vi "SetAnalogTrigger.vi"(8 "error in (no error)":errorcluster, 10 "Trigger Config":T1={"Channel"=enum."chn B", "Edge"=0, "Level[V]"=0.5} {"Edge" items=["RISING", "FALLING", "ANY"]}, 11 "reference in":refnum<k24>) -> (0 "error out":errorcluster, 3 "reference out":refnum<k24>)   [LabVIEW 2019, in "LabNation Scope Driver.lvlib"]
doc: "Sets the Trigger."
uses:
  LabNation Scope Driver.lvlib
  Typedef/TriggerData.ctl
  Typedef/Channel Selection.ctl
  Typedef/Edge.ctl
  C:/Program Files (x86)/LabNation/SmartScope/DeviceInterface.dll
  Program Files (x86)/LabNation/SmartScope/DeviceInterface.dll
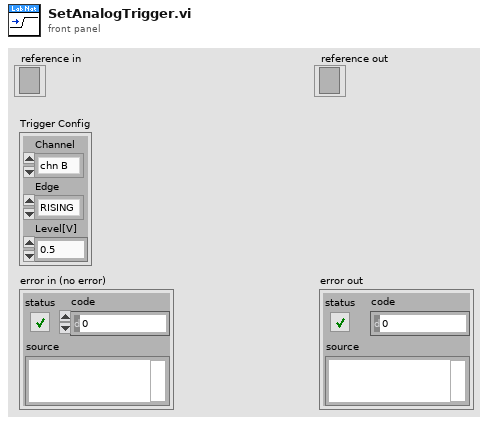
[diagram p1: front panel]
types:
  T1 = typedef "LabNation Scope Driver.lvlib/TriggerData.ctl" = cluster{"Channel":T2, "Edge":T3, "Level[V]":sgl}
  T2 = typedef "LabNation Scope Driver.lvlib/Channel Selection.ctl" = enum16{"chn A", "chn B"}
  T3 = typedef "LabNation Scope Driver.lvlib/Edge.ctl" = i32
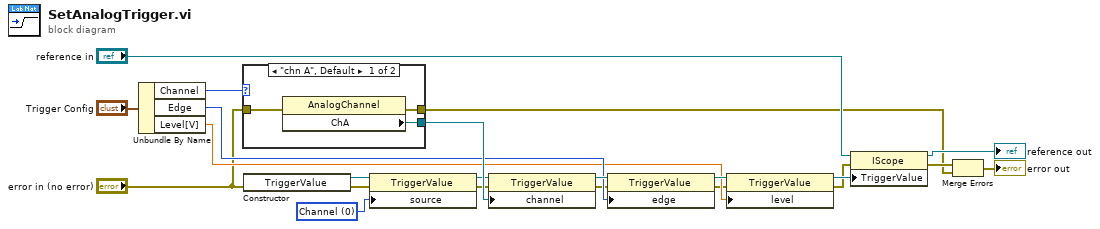
[diagram p0: block diagram]
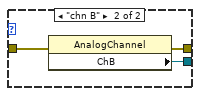
[diagram p2: hidden frame]
diagram:
  w19 = 0 items=["Channel", "External"] ("source")
  n1 = Unbundle By Name("Trigger Config") -> ("Channel"=w11:T2, "Edge"=w10:T3, "Level[V]"=w9:sgl)
  n2 = case shown="\"chn A\", Default" w11 {
    tunnel: [w25 w28] -> w22
    tunnel: "error in (no error)" -> [w23 w27]
    tunnel: [w24 w26] -> w1
    frame "chn A", Default {
      n3 = property class="AnalogChannel"(error in=w23) -> (error out=w24:errorcluster, "ChA"=w25:refnum<k24>)  [unwired: 1 in, 1 out]
    }
    frame "chn B" {
      n4 = property class="AnalogChannel"(error in=w27) -> (error out=w26:errorcluster, "ChB"=w28:refnum<k24>)  [unwired: 1 in, 1 out]
    }
  }
  n5 = constructor class="TriggerValue"(error in="error in (no error)") -> (reference out=w20:refnum<k24>, error out=w8:errorcluster)  [unwired: 2 in, 1 out]
  n6 = property class="TriggerValue"(reference=w20, error in=w8, "source"=w19) -> (reference out=w18:refnum<k24>, error out=w7:errorcluster)
  n7 = property class="TriggerValue"(reference=w18, error in=w7, "channel"=w22) -> (reference out=w17:refnum<k24>, error out=w6:errorcluster)
  n8 = property class="TriggerValue"(reference=w17, error in=w6, "edge"=w10) -> (reference out=w16:refnum<k24>, error out=w5:errorcluster)
  n9 = property class="TriggerValue"(reference=w16, error in=w5, "level"=w9) -> (reference out=w21:refnum<k24>, error out=w4:errorcluster)
  n10 = property class="IScope"(reference="reference in", error in=w4, "TriggerValue"=w21) -> (reference out=→"reference out":refnum<k24>, error out=w13:errorcluster)
  n11 = Merge Errors(w13, w1) -> (→"error out":errorcluster)
